vi "Fetch List Items From Lookup (SubVI).vi"(3 "error IN":errorcluster, 5 "Query":string) -> (0 "error OUT":errorcluster, 2 "recordset data":string[][](array[string]))   [LabVIEW 2015]
uses:
  <vilib>/addons/database/Connection.llb/DB Tools Open Connec (Path).vi
  <vilib>/addons/database/Connection.llb/Conn Execute.vi
  <vilib>/addons/database/Recordset.llb/Rec Destroy - Connection.vi
  <vilib>/addons/database/NI_Database_API.lvlib
panel:
  out "App.Dir":path
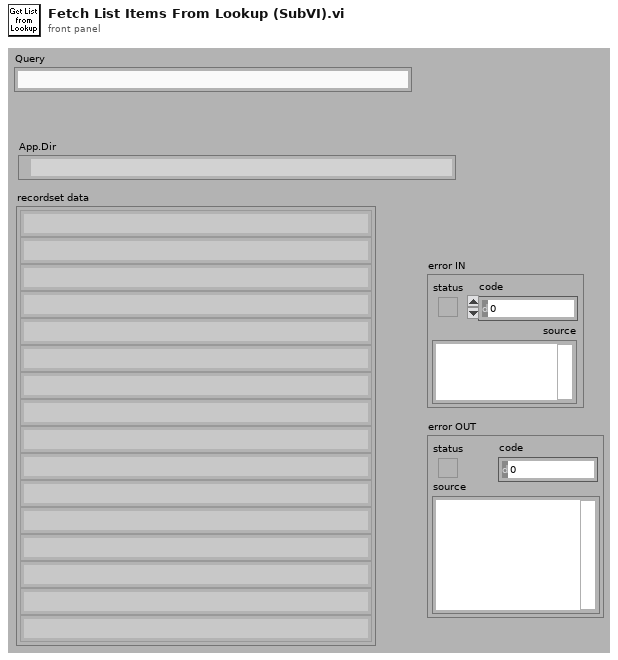
[diagram p1: front panel]
types:
  T1 = enum32{"invalid app kind", "Development System", "Run Time System", "Student Edition", "Embedded LabVIEW", "Evaluation", "Custom"}
  T2 = typedef "NI_Database_API.lvlib/Conn ObjectReference.ctl" = refnum<k1>
  T3 = typedef "NI_Database_API.lvlib/Rec ObjectReference.ctl" = refnum<k1>
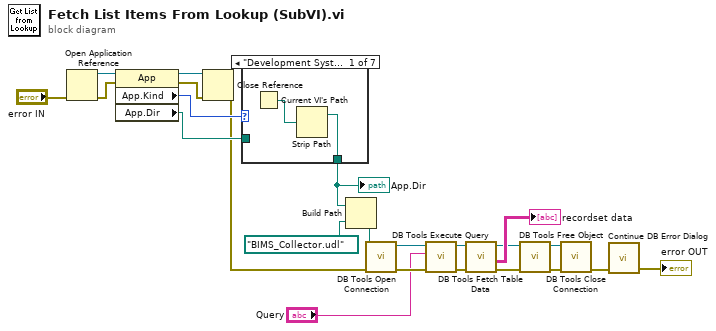
[diagram p0: block diagram]
diagram:
  n1 = Open Application Reference(8:"error IN") -> (0:w8:errorcluster, 3:w9:refnum<vi>)  [unwired: 3 out]
  n2 = property class="App"(reference=w9, error in=w8) -> (reference out=w7:refnum<vi>, error out=w6:errorcluster, "App.Kind"=w5:T1, "App.Dir"=w4:path)
  n3 = Close Reference(reference=w7, error in (no error)=w6) -> (error out=w1:errorcluster)
  n4 = case shown="\"Development System\"" w5 {
    tunnel: [w24 w26 w27 w28 w29 w30 w31] -> w3
    tunnel: w4 -> [_ w26 w27 w28 w29 w30 w31]
    frame "Development System" {
      n5 = Current VI's Path() -> (path=w25:path)
      n6 = Strip Path(path=w25) -> (stripped path=w24:path)  [unwired: 1 out]
    }
    frame "Run Time System" {
    }
    frame "Student Edition" {
    }
    frame "Embedded LabVIEW" {
    }
    frame "Evaluation" {
    }
    frame "Custom" {
    }
    frame "invalid app kind" {
    }
  }
  "App.Dir" <- w3
  n7 = Build Path(base path=w3, name or relative path=path "BIMS_Collector.udl" ("connectString")) -> (appended path=w11:path)
  n8 = call-poly <vilib>:"DB Tools Open Connection.vi"("error in (no error)"=w1, "connection information"=w11) -> ("error out"=w17:errorcluster, "connection reference"=w15:T2)  [unwired: 3 in, 3 out]
  n9 = call-poly <vilib>:"DB Tools Execute Query.vi"("error in (no error)"=w17, "SQL query"="Query", "connection reference"=w15) -> ("error out"=w18:errorcluster, "recordset reference"=w14:T3)  [unwired: 1 in, 4 out]
  n10 = call <vilib>:"DB Tools Fetch Table Data.vi"("error in (no error)"=w18, "recordset reference"=w14) -> ("error out"=w19:errorcluster, "recordset data"=→"recordset data":string[][], "recordset reference out"=w13:T3)  [unwired: 3 out]
  n11 = call-poly <vilib>:"DB Tools Free Object.vi"("error in (no error)"=w19, "recordset reference"=w13) -> ("error out"=w20:errorcluster, "connection reference"=w16:T2)  [unwired: 8 out]
  n12 = call <vilib>:"DB Tools Close Connection.vi"("error in (no error)"=w20, "connection reference"=w16) -> ("error out"=w22:errorcluster)  [unwired: 5 out]
  n13 = call "Continue DB Error Dialog.vi"("error in (no error)"=w22) -> ("error out"=→"error OUT":errorcluster)  [unwired: 3 in, 2 out]
